vi "Acquired points counter.vi"(0 "Logging queue element":T1={"Imaging Protocol"=enum."Live Imaging", "Number of Trials"=0, "Frame Size"=512, "# Averaged frames"=0, "Dwell time (us)"=0.0, "Index of Z-plane"=0, "Timelapse?"=FALSE, "Logging process is active"=FALSE, "Speed logging enabled"=FALSE, "tdms file ref"=refnum, "path"=path "", "Trial Number"=0, "Expected # points acquired"=FALSE, "Manually stopped"=FALSE, "Last trial"=FALSE, "Ch0 data"=[], "Ch1 data"=[], "Image Time"=[], "Continuous Time"=[], "Points acquired"={"Ch0 last trial"=0, "Ch1 last trial"=0, "All trials"=0}, "HW Timings File"=refnum} {"Frame Size" items=["100X100"=100, "128X128"=128, "200X200"=200, "256X256"=256, "512X512"=512, "1024x1024"=1024, "2048x2048"=2048]; "Dwell time (us)" format="%#.6g"}, 5 "Raw Data Array":T5, 7 "Number of samples to be acquired (points in frame x Ch. x Av.)":u64, 11 "error in":errorcluster, 12 "Initial reset":bool, 13 "Max allowed trial length (sec)":dbl=15.0 format="%#_13g") -> (4 "Logging queue element":T1={"Imaging Protocol"=enum."Live Imaging", "Number of Trials"=0, "Frame Size"=512, "# Averaged frames"=0, "Dwell time (us)"=0.0, "Index of Z-plane"=0, "Timelapse?"=FALSE, "Logging process is active"=FALSE, "Speed logging enabled"=FALSE, "tdms file ref"=refnum, "path"=path "", "Trial Number"=0, "Expected # points acquired"=FALSE, "Manually stopped"=FALSE, "Last trial"=FALSE, "Ch0 data"=[], "Ch1 data"=[], "Image Time"=[], "Continuous Time"=[], "Points acquired"={"Ch0 last trial"=0, "Ch1 last trial"=0, "All trials"=0}, "HW Timings File"=refnum} {"Frame Size" items=["100X100"=100, "128X128"=128, "200X200"=200, "256X256"=256, "512X512"=512, "1024x1024"=1024, "2048x2048"=2048]; "Dwell time (us)" format="%#.6g"}, 8 "Expected number of funct.acq points acquired on both channels":bool, 10 "Live imaging stopped":bool, 15 "error out":errorcluster)   [LabVIEW 2017]
uses:
  Typedefs/Data arrays cluster.ctl
  Typedefs/Logging queue element.ctl
  Typedefs/Imaging Protocols enum.ctl
  Typedefs/Frame Size.ctl
  Typedefs/Acquired points count.ctl
  Typedefs/Read Write Enum.ctl
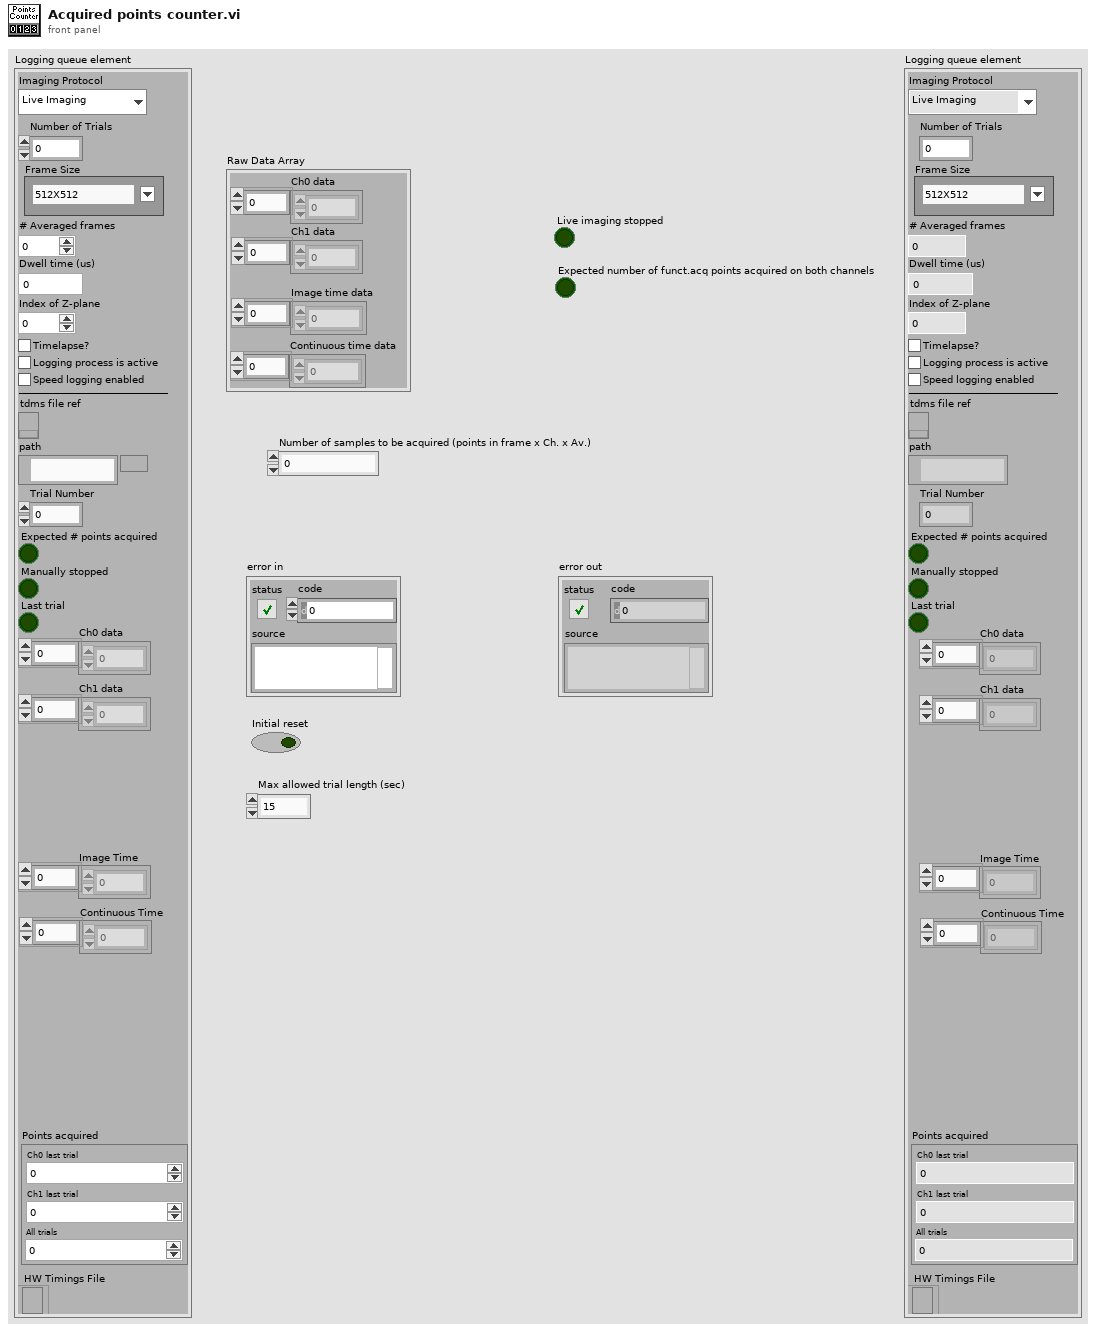
[diagram p1: front panel]
types:
  T1 = typedef "Logging queue element.ctl" = cluster{"Imaging Protocol":T2, "Number of Trials":u16, "Frame Size":T3, "# Averaged frames":u16, "Dwell time (us)":dbl, "Index of Z-plane":i32, "Timelapse?":bool, "Logging process is active":bool, "Speed logging enabled":bool, "tdms file ref":refnum<k34>, "path":path, "Trial Number":i32, "Expected # points acquired":bool, "Manually stopped":bool, "Last trial":bool, "Ch0 data":u32[], "Ch1 data":u32[], "Image Time":u64[], "Continuous Time":u64[], "Points acquired":T4, "HW Timings File":refnum<file>}
  T2 = typedef "Imaging Protocols enum.ctl" = enum16{"AOL Z-Stack", "Motor Z Stack", "Functional Acquisition", "Single Plane Acquisition", "Volume Acquisition", "Live Imaging", "Live Plane Imaging", "Live Volume Imaging"}
  T3 = typedef "Frame Size.ctl" = u16
  T4 = typedef "Acquired points count.ctl" = cluster{"Ch0 last trial":u64, "Ch1 last trial":u64, "All trials":u64}
  T5 = typedef "Data arrays cluster.ctl" = cluster{"Ch0 data":u32[], "Ch1 data":u32[], "Image time data":u64[], "Continuous time data":u64[]}
  T6 = typedef "Read Write Enum.ctl" = enum16{"Read", "Write"}
  T7 = cluster{u64, "Number of samples to be acquired (points in frame x Ch. x Av.)":u64, "Trial Number":i32}
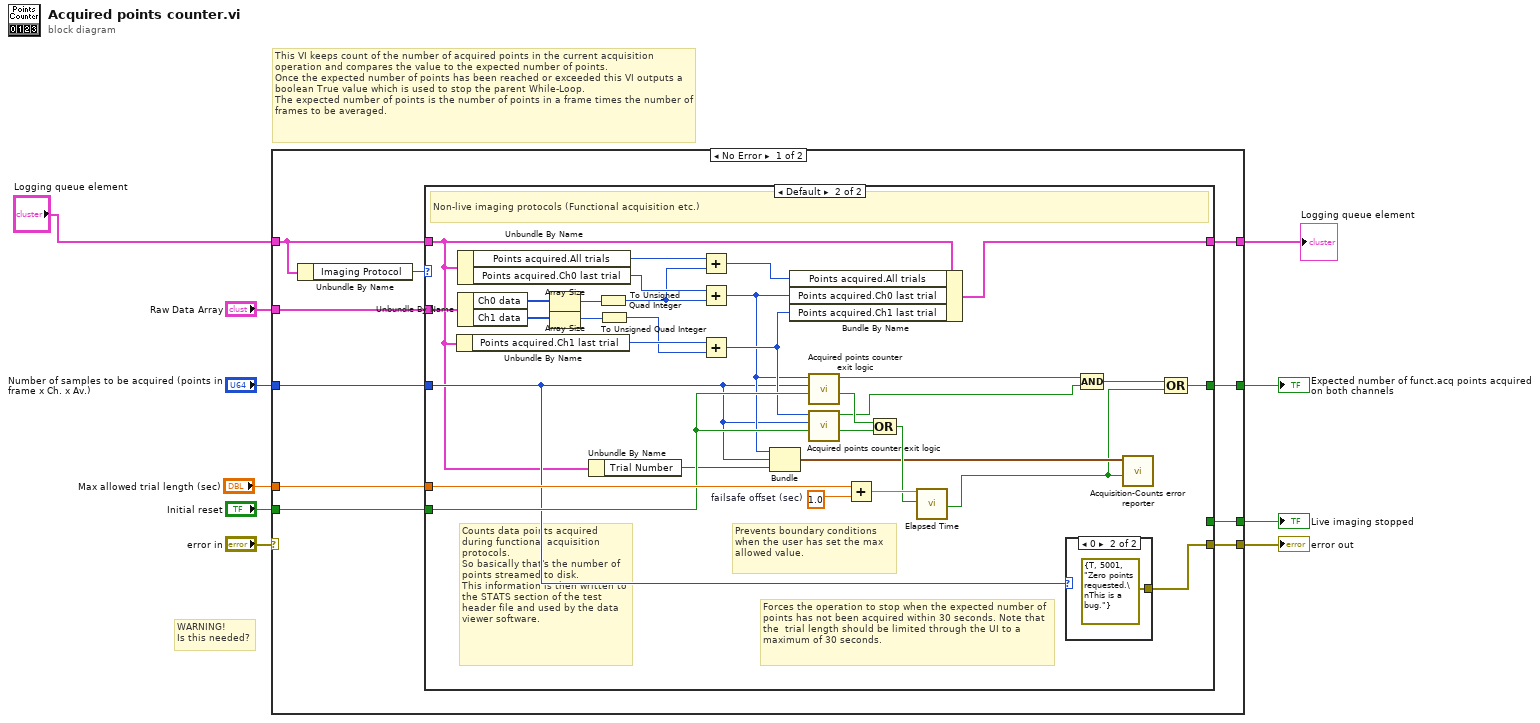
[diagram p0: block diagram]
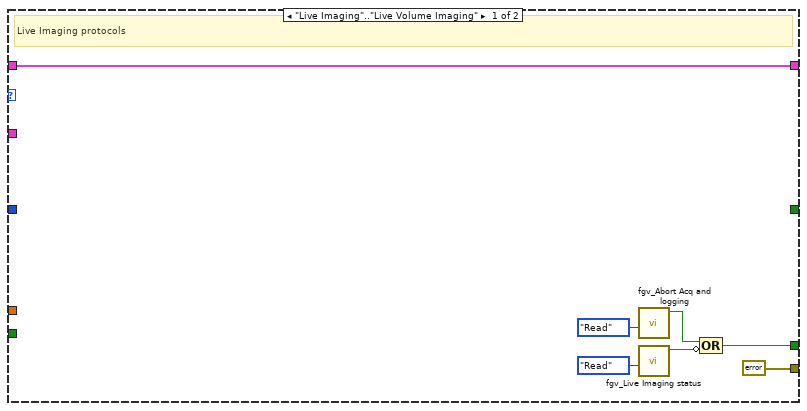
[diagram p2: hidden frame]
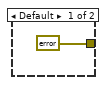
[diagram p3: hidden frame]
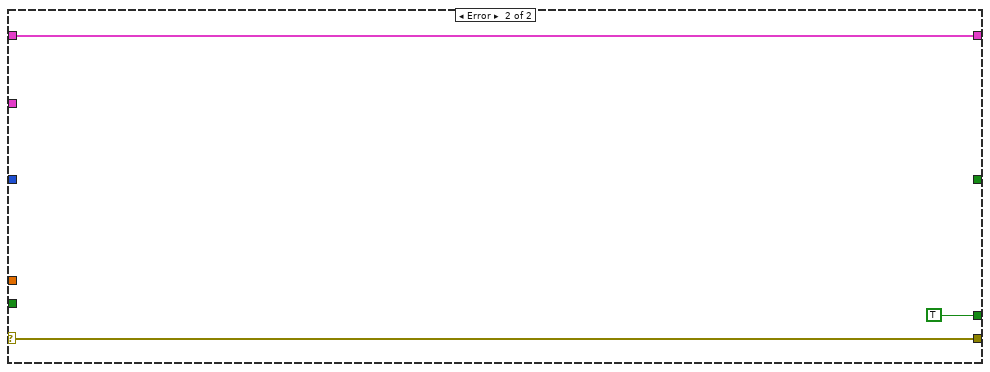
[diagram p4: hidden frame]
diagram:
  # "WARNING!\nIs this needed?"
  # "This VI keeps count of the number of acquired points in the current acquisition operation and compares the value to the expected number of points. \nOnce the expected number of points has been reached or exceeded this VI outputs a boolean True value which is used to stop the parent While-Loop.\nThe expected number of points is the number of points in a frame times the number of frames to be averaged."
  n1 = case shown="No Error" "error in" {
    selector: "error in" -> [_ w63]
    tunnel: "Number of samples to be acquired (points in frame x Ch. x Av.)" -> [w20 _]
    tunnel: [w19 _] -> w6
    tunnel: "Raw Data Array" -> [w13 _]
    tunnel: [w17 TRUE] -> w9
    tunnel: "Logging queue element" -> [w12 w61]
    tunnel: [w14 w63] -> w7
    tunnel: "Initial reset" -> [w16 _]
    tunnel: "Max allowed trial length (sec)" -> [w15 _]
    tunnel: [w11 w61] -> w1
    frame No Error {
      n2 = Unbundle By Name(w12) -> ("Imaging Protocol"=w18:T2)
      n3 = case shown="Default" w18 {
        tunnel: w20 -> [_ w32]
        tunnel: [_ w58] -> w19
        tunnel: [w27 _] -> w17
        tunnel: w16 -> [_ w50]
        tunnel: w15 -> [_ w57]
        tunnel: [errorcluster {"status"=FALSE, "code"=0, "source"=""} ("error out") w54] -> w14
        tunnel: w13 -> [_ w42]
        tunnel: w12 -> [w21 w29]
        tunnel: [w21 w38] -> w11
        frame "Live Imaging".."Live Volume Imaging" {
          # "Live Imaging protocols"
          n4 = call "fgv_Abort Acq and logging.vi"("Function"=Read_Write_Enum."Read") -> ("Abort acquisition"=w23:bool)  [unwired: 9 in, 1 out]
          n5 = call "fgv_Live Imaging status.vi"("Function"=Read_Write_Enum."Read") -> ("Live Imaging?"=w25:bool)  [unwired: 9 in, 1 out]
          n6 = Compound Arithmetic op=OR(w23, invert w25) -> (w27:bool)
        }
        frame Default {
          w55 = 1.0  # failsafe offset (sec)
          # "Counts data points acquired during functional acquisition protocols.\nSo basically that's the number of points streamed to disk.\nThis information is then written to the STATS section of the test header file and used by the data viewer software."
          # "Prevents boundary conditions when the user has set the max allowed value."
          # "Forces the operation to stop when the expected number of points has not been acquired within 30 seconds. Note that the  trial length should be limited through the UI to a maximum of 30 seconds."
          # "Non-live imaging protocols (Functional acquisition etc.)"
          n7 = Unbundle By Name(w29) -> ("Points acquired.Ch1 last trial"=w40:u64)
          n8 = Unbundle By Name(w29) -> ("Points acquired.All trials"=w37:u64, "Points acquired.Ch0 last trial"=w41:u64)
          n9 = Unbundle By Name(w42) -> ("Ch0 data"=w45:u32[], "Ch1 data"=w44:u32[])
          n10 = Array Size(array=w45) -> (size(s)=w46:i32)
          n11 = Array Size(array=w44) -> (size(s)=w43:i32)
          n12 = Unbundle By Name(w29) -> ("Trial Number"=w28:i32)
          n13 = To Unsigned Quad Integer(1:w46) -> (0:w35:u64)
          n14 = To Unsigned Quad Integer(1:w43) -> (0:w34:u64)
          n15 = Add(x=w37, y=w35) -> (x+y=w36:u64)
          n16 = Add(x=w41, y=w35) -> (x+y=w33:u64)
          n17 = Add(x=w40, y=w34) -> (x+y=w39:u64)
          n18 = Bundle(w33, "Number of samples to be acquired (points in frame x Ch. x Av.)"=w32, "Trial Number"=w28) -> (w31:T7)  [unwired: 1 in]
          n19 = Bundle By Name(cluster=w29, "Points acquired.All trials"=w36, "Points acquired.Ch0 last trial"=w33, "Points acquired.Ch1 last trial"=w39) -> (w38:T1)
          n20 = call "Acquired points counter exit logic.vi"("Initial reset"=w50, "Number of samples to be acquired in each trial (i.e. Target samples)"=w32, "Running Count (current trial)"=w33) -> ("Reset fail-safe timeout"=w53:bool, "Stop acquisition loop"=w48:bool)  [unwired: 7 in]
          n21 = call "Acquired points counter exit logic.vi"("Initial reset"=w50, "Number of samples to be acquired in each trial (i.e. Target samples)"=w32, "Running Count (current trial)"=w39) -> ("Reset fail-safe timeout"=w51:bool, "Stop acquisition loop"=w49:bool)  [unwired: 7 in]
          n22 = Add(x=w57, y=w55) -> (x+y=w56:dbl)
          n23 = Compound Arithmetic op=OR(w53, w51) -> (w52:bool)
          n24 = call "Elapsed Time"("Time Target (s)"=w56, "Reset"=w52) -> ("Time has Elapsed"=w30:bool)  [unwired: 10 in, 7 out]
          n25 = case shown="0" w32 {
            tunnel: [errorcluster {"status"=FALSE, "code"=0, "source"=""} ("f") errorcluster {"status"=TRUE, "code"=5001, "source"="Zero points requested.\nThis is a bug."} ("error out")] -> w54
            frame Default {
            }
            frame 0 {
            }
          }
          n26 = Compound Arithmetic op=AND(w48, w49) -> (w47:bool)
          n27 = call "Acquisition-Counts error reporter.vi"("Timed out waiting for expected number of acquisition points"=w30, "Counts cluster"=w31) -> ()  [unwired: 10 in]
          n28 = Compound Arithmetic op=OR(w47, w30) -> (w58:bool)
        }
      }
    }
    frame Error {
    }
  }
  "Expected number of funct.acq points acquired on both channels" <- w6
  "error out" <- w7
  "Live imaging stopped" <- w9
  "Logging queue element" <- w1
